vi "Method.vi"(4 "Value":refnum<class "Abs_Double Float.lvclass">) -> (1 "Result":refnum<class "Abs_Double Float.lvclass">)   [LabVIEW 2021, in "Invert_CPLX_DBL.lvclass"]
uses:
  Invert_CPLX_DBL.lvclass
  Abs_Types/Double Float/Abs_Double Float.lvclass
  C:/TSA/LV_Abstract/Source/Functions/Support/Function/One Terminal/DBL/AbsFunc_One Term_DBL.lvclass
  C:/Program Files (x86)/National Instruments/LabVIEW 2021/vi.lib/TSA/Abstract Data Classes/Abs_Types/Double Float/Abs_Double Float.lvclass
  Support/Function/One Terminal/DBL/AbsFunc_One Term_DBL.lvclass/AbsFunc_One Term_DBL.ctl
  Support/Function/One Terminal/DBL/Properties/Write Numeric A.vi
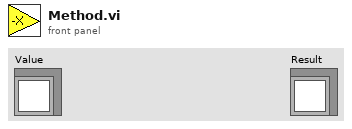
[diagram p1: front panel]
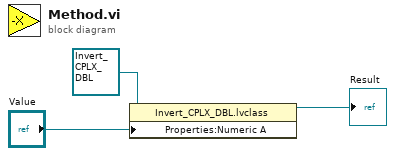
[diagram p0: block diagram]
diagram:
  n1 = property class="Invert_CPLX_DBL.lvclass"(reference=refnum<class "Invert_CPLX_DBL.lvclass"> refnum ("Invert_DBL.lvclass"), "Properties:Numeric A"="Value") -> (reference out=→"Result":refnum<class "Invert_CPLX_DBL.lvclass">)  [unwired: 1 in, 1 out]
